vi "QControl Creator Main.vi"(6 "CreatorComplete":refnum<user-event>, 8 "error in (no error)":errorcluster, 9 "StatusUpdate":refnum<user-event>, 10 "New QControl Information":T1, 11 "App Refnum":refnum<vi>) -> (0 "error out":errorcluster, 3 "CreatorRefnum":refnum<vi>)   [LabVIEW 2015, in "QControl Creation.lvclass"]
doc: "<b> </b> <b> </b>\n©2016 Q Software Innovations, LLC (QSI)\nwritten by Quentin Alldredge\nproduced in LabVIEW 2015\n\nsupport@qsoftwareinnovations.com\nwww.qsoftwareinnovations.com\n\nAll rights reserved.\n\nRedistribution and use in source and binary forms, with or without modification, are permitted provided that the following conditions are met:\n\n * Redistributions of source code must retain the above copyright notice, this list of conditions and the following disclaimer.\n * Redistributions in binary form must reproduce the above copyright notice, this list of conditions and the following disclaimer in the documentation and/or other materials provided with the distribution.\n * Neither the name of Q Software Innovations, LLC. nor the names of its contributors may be used to endorse or promote products derived from this software without specific prior written permission.\n\nTHIS SOFTWARE IS PROVIDED BY THE COPYRIGHT HOLDERS AND CONTRIBUTORS \"AS IS\" AND ANY EXPRESS OR IMPLIED WARRANTIES, INCLUDING, BUT NOT LIMITED TO, THE IMPLIED WARRANTIES OF MERCHANTABILITY AND FITNESS FOR A PARTICULAR PURPOSE ARE DISCLAIMED. IN NO EVENT SHALL THE COPYRIGHT OWNER OR CONTRIBUTORS BE LIABLE FOR ANY DIRECT, INDIRECT, INCIDENTAL, SPECIAL, EXEMPLARY, OR CONSEQUENTIAL DAMAGES (INCLUDING, BUT NOT LIMITED TO, PROCUREMENT OF SUBSTITUTE GOODS OR SERVICES; LOSS OF USE, DATA, OR PROFITS; OR BUSINESS INTERRUPTION) HOWEVER CAUSED AND ON ANY THEORY OF LIABILITY, WHETHER IN CONTRACT, STRICT LIABILITY, OR TORT (INCLUDING NEGLIGENCE OR OTHERWISE) ARISING IN ANY WAY OUT OF THE USE OF THIS SOFTWARE, EVEN IF ADVISED OF THE POSSIBILITY OF SUCH DAMAGE."
uses:
  QControl Creation.lvclass
  New QControl Information.ctl
  QControl Creation.lvclass/QControl Creation.ctl
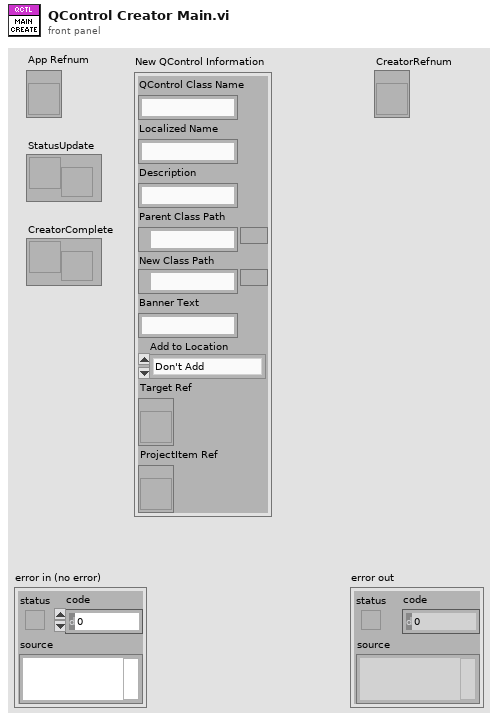
[diagram p1: front panel]
types:
  T1 = typedef "QControl Creation.lvclass/New QControl Information.ctl" = cluster{"QControl Class Name":string, "Localized Name":string, "Description":string, "Parent Class Path":path, "New Class Path":path, "Banner Text":string, "Add to Location":enum16{"Don't Add", "To Target", "To Project Item"}, "Target Ref":refnum<vi>, "ProjectItem Ref":refnum<vi>}
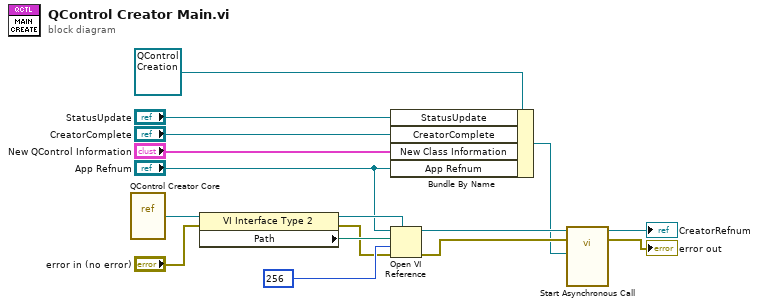
[diagram p0: block diagram]
diagram:
  n1 = vi-ref "QControl Creator Core.vi"() -> (w16:refnum<vi>)
  n2 = property class="VI Interface Type 2"(reference=w16, error in="error in (no error)") -> (reference out=w13:refnum<vi>, error out=w4:errorcluster, "Path"=w15:path)
  n3 = Bundle By Name(cluster=refnum<class "QControl Creation.lvclass"> refnum ("QControl Creation in"), "StatusUpdate"="StatusUpdate", "CreatorComplete"="CreatorComplete", "New Class Information"="New QControl Information", "App Refnum"="App Refnum") -> (w1:refnum<class "QControl Creation.lvclass">)
  n4 = Open VI Reference(type specifier VI Refnum (for type only)=w13, application reference (local)="App Refnum", vi path=w15, options=256, error in (no error)=w4) -> (vi reference=w12:refnum<vi>, error out=w2:errorcluster)  [unwired: 1 in]
  n5 = call-by-ref "Start Asynchronous Call"(reference=w12, error in=w2, "QControl Creation in"=w1) -> (reference out=→"CreatorRefnum":refnum<vi>, error out=→"error out":errorcluster)  [unwired: 10 in, 1 out]
